vi "Set Dev Notice Call Back.vi"(8 "error in (no error)":errorcluster, 9 "rmvcallback":cluster{}, 10 "addcallback":cluster{}, 11 "ppara":u32) -> (0 "error out":errorcluster, 3 "ppara out":u32)   [LabVIEW 2021, in "vmmso.lvlib"]
doc: "DLL_API void WINAPI SetDevNoticeCallBack(void* ppara, AddCallBack addcallback, RemoveCallBack rmvcallback);"
uses:
  vmmso.lvlib
  vmmso.dll
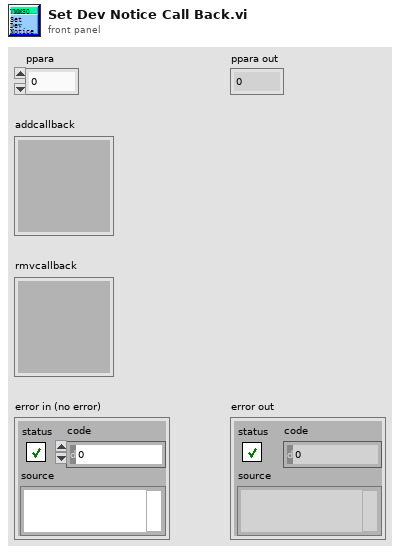
[diagram p1: front panel]
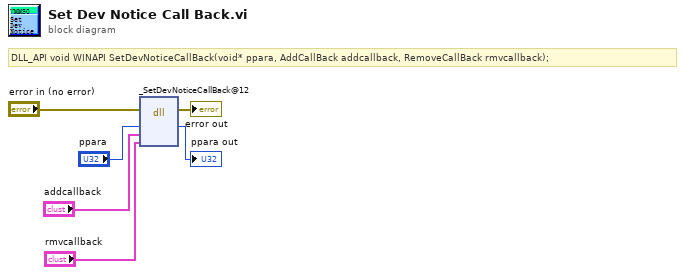
[diagram p0: block diagram]
diagram:
  # "DLL_API void WINAPI SetDevNoticeCallBack(void* ppara, AddCallBack addcallback, RemoveCallBack rmvcallback);"
  n1 = dll-call lib="O:/MSO/library/demo-Labview/vmmso/vmmso.*" fn="_SetDevNoticeCallBack@12"(error in="error in (no error)", "ppara"="ppara", "addcallback"="addcallback", "rmvcallback"="rmvcallback") -> (error out=→"error out":errorcluster, "ppara"=→"ppara out":u32)  [unwired: 5 in, 1 out]
